vi "Send Active Event.vi"(8 "error in (no error)":errorcluster, 11 "QMenu Class in":refnum<class "QMenu Class.lvclass">) -> (0 "error out":errorcluster, 3 "QMenu Class out":refnum<class "QMenu Class.lvclass">)   [LabVIEW 2020, in "QTab.lvlib" / "QMenu Class.lvclass"]
uses:
  QMenu Class.lvclass
  QMenu Class.lvclass/QMenu Class.ctl
  Active Event Data.ctl
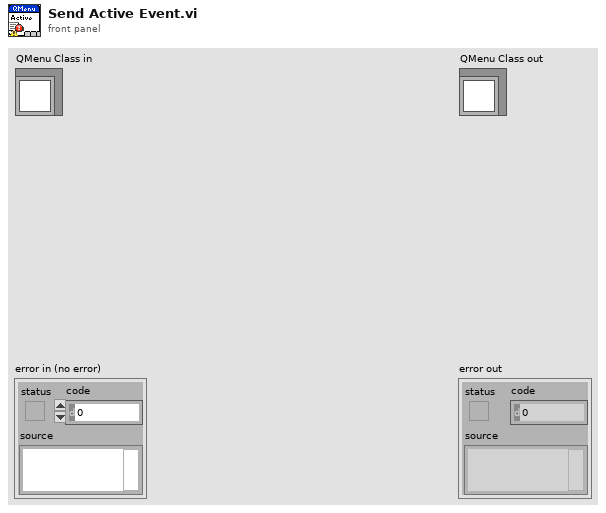
[diagram p1: front panel]
types:
  T1 = typedef "QTab.lvlib/QMenu Class.lvclass/Active Event Data.ctl" = cluster{"Index":i32, "Label":string}
  T2 = typedef "QTab.lvlib/QMenu Class.lvclass/Button Attribute.ctl" = cluster{"Label":string, "Button Text":string, "Closable":bool, "Draggable":bool}
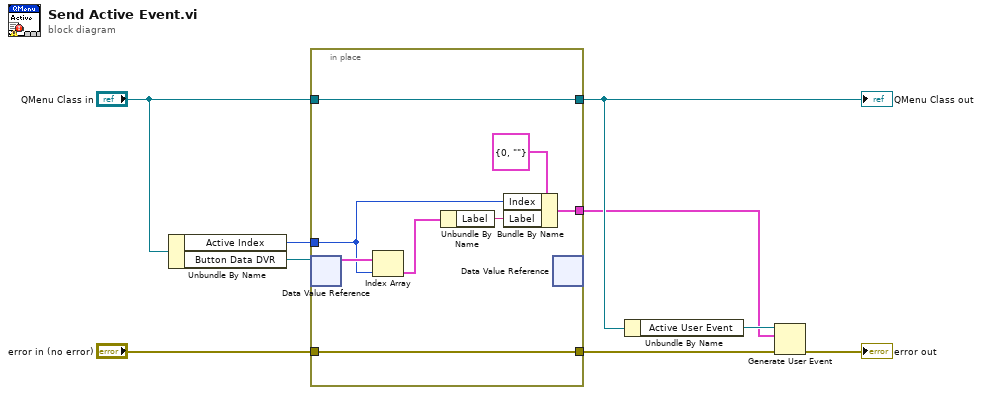
[diagram p0: block diagram]
diagram:
  n1 = Unbundle By Name("QMenu Class in") -> ("Active Index"=w4:i32, "Button Data DVR"=w8:refnum<data-value>)
  n2 = in-place {
    in-place-border: w4 -> [w14]
    in-place-border: "error in (no error)" -> [w11]
    in-place-border: "QMenu Class in" -> [w17]
    in-place-border: [w17] -> w5
    in-place-border: [w16] -> w1
    in-place-border: [w11] -> w2
    n3 = in-place-dvr #1(w8) -> (w15:T2[])  [unwired: 1 out]
    n4 = Index Array(array=w15, index=w14) -> (element=w13:T2)
    n5 = Unbundle By Name(w13) -> ("Label"=w12:string)
    n6 = Bundle By Name(cluster=T1 {"Index"=0, "Label"=""} ("event data"), "Index"=w14, "Label"=w12) -> (w16:T1)
    n7 = in-place-dvr #1() -> ()  [unwired: 1 in, 2 out]
  }
  "QMenu Class out" <- w5
  n8 = Unbundle By Name(w5) -> ("Active User Event"=w3:refnum<user-event>)
  n9 = Generate User Event(user event=w3, event data cluster=w1, error in=w2) -> (error out=→"error out":errorcluster)  [unwired: 1 in, 1 out]
